vi "CheckVeriStandVersionMatchesLabVIEW.vi"(8 "error in (no error)":errorcluster, 11 "Target (localhost)":refnum<k21>="localhost") -> (0 "error out":errorcluster, 3 "versions match?":bool)   [LabVIEW 2027, in "VeriStandTestUtilities.lvlib"]
uses:
  VeriStandTestUtilities.lvlib
  <vilib>/nisyscfg/Get Installed Components.vi
  <vilib>/nisyscfg/Close (System).vi
  <vilib>/regexp/Match Regular Expression.xnode
  <vilib>/nisyscfg/nisyscfg.lvlib
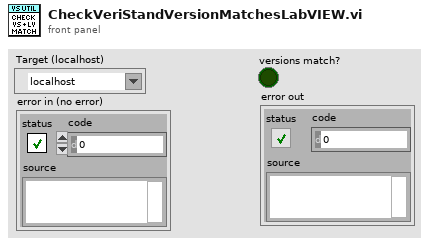
[diagram p1: front panel]
types:
  T1 = typedef "nisyscfg.lvlib/Software 1.2.ctl" = cluster{"title":string, "description":string, "ID":string, "version":string, "component type":T2}
  T2 = typedef "nisyscfg.lvlib/Component Type.ctl" = u32
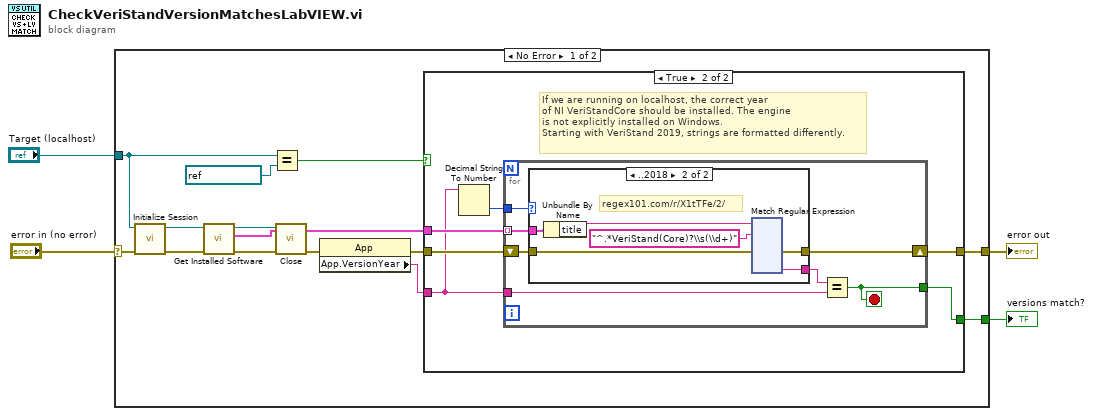
[diagram p0: block diagram]
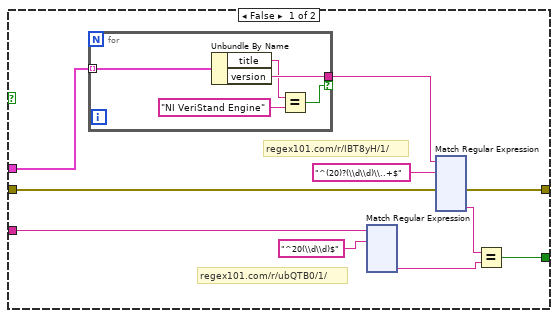
[diagram p2: hidden frame]
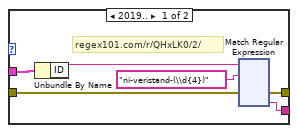
[diagram p3: hidden frame]
diagram:
  n1 = case shown="No Error" "error in (no error)" {
    selector: "error in (no error)" -> [w15 w537]
    tunnel: [w18 _] -> w4
    tunnel: "Target (localhost)" -> [w16 _]
    tunnel: [w14 w537] -> w1
    frame No Error {
      n2 = call <vilib>:"Initialize Session.vi"("error in (no error)"=w15, "Target (localhost)"=w16) -> ("error out"=w10:errorcluster, "Session out"=w13:refnum<k21>)  [unwired: 8 in]
      n3 = call-poly <vilib>:"Get Installed Software.vi"("error in (no error)"=w10, "Session in"=w13) -> ("error out"=w11:errorcluster, "Software Components"=w8:T1[], "Session out"=w12:refnum<k21>)  [unwired: 7 in]
      n4 = Equal?(x=w16, y=refnum<k21> "localhost" ("Target (localhost)")) -> (x = y?=w9:bool)
      n5 = call-poly <vilib>:"Close.vi"("error in (no error)"=w11, "Session in"=w12) -> ("error out"=w6:errorcluster)  [unwired: 9 in]
      n6 = property class="App"(error in=w6) -> (error out=w7:errorcluster, "App.VersionYear"=w5:string)  [unwired: 1 in, 1 out]
      n7 = case shown="True" w9 {
        tunnel: [w25 w277] -> w18
        tunnel: [w23 w275] -> w14
        tunnel: w8 -> [w28 w278]
        tunnel: w7 -> [w24 w276]
        tunnel: w5 -> [w21 w273]
        frame False {
          # "regex101.com/r/ubQTB0/1/"
          # "regex101.com/r/IBT8yH/1/"
          n8 = for {
            tunnel: w28 -> [w33] mode=indexing
            tunnel: [w31] -> w27 if=w30
            n9 = Unbundle By Name(w33) -> ("title"=w29:string, "version"=w31:string)
            n10 = Equal?(x=w29, y="NI VeriStand Engine") -> (x = y?=w30:bool)
          }
          n11 = xnode "Match Regular Expression"("input string"=w21, "regular expression"="^20(\\d\\d)$" ("y")) -> ("submatch 1"=w19:string)  [unwired: 4 in, 5 out]
          n12 = xnode "Match Regular Expression"("input string"=w27, "regular expression"="^(20)?(\\d\\d)\\..+$" ("y"), "error in"=w24) -> ("error out"=w23:errorcluster, "submatch 2"=w22:string)  [unwired: 3 in, 5 out]
          n13 = Equal?(x=w22, y=w19) -> (x = y?=w25:bool)
        }
        frame True {
          # "If we are running on localhost, the correct year\nof NI VeriStandCore should be installed. The engine\nis not explicitly installed on Windows.\nStarting with VeriStand 2019, strings are formatted differently."
          n14 = Decimal String To Number(string=w273) -> (number=w274:i32)  [unwired: 2 in, 1 out]
          n15 = for {
            tunnel: w278 -> [w282] mode=indexing
            tunnel: w273 -> [w285]
            tunnel: [w284] -> w277
            shift-right: [w279] -> w275
            shift-left: w276 -> [w280]
            tunnel: w274 -> [w283]
            stop <- w284 stop-if-true
            n16 = case shown="..2018" w283 {
              tunnel: w282 -> [w289 w414]
              tunnel: [w288 w413] -> w281
              tunnel: w280 -> [w287 w412]
              tunnel: [w286 w411] -> w279
              frame 2019.. {
                # "regex101.com/r/QHxLK0/2/"
                n17 = Unbundle By Name(w289) -> ("ID"=w290:string)
                n18 = xnode "Match Regular Expression"("input string"=w290, "regular expression"="ni-veristand-(\\d{4})" ("y"), "error in"=w287) -> ("error out"=w286:errorcluster, "submatch 1"=w288:string)  [unwired: 3 in, 4 out]
              }
              frame ..2018 {
                # "regex101.com/r/X1tTFe/2/"
                n19 = Unbundle By Name(w414) -> ("title"=w415:string)
                n20 = xnode "Match Regular Expression"("input string"=w415, "regular expression"="^.*VeriStand(Core)?\\s(\\d+)" ("y"), "error in"=w412) -> ("error out"=w411:errorcluster, "submatch 2"=w413:string)  [unwired: 3 in, 5 out]
              }
            }
            n21 = Equal?(x=w281, y=w285) -> (x = y?=w284:bool)
          }
        }
      }
    }
    frame Error {
    }
  }
  "versions match?" <- w4
  "error out" <- w1
